vi "Register for Sequence Complete Event.vi"(8 "error in (no error)":errorcluster, 10 "Sequence Names":string[](array[string]), 11 "Session Ref in":T2) -> (0 "error out":errorcluster, 1 "Event Registration Refnum":refnum<event-registration>, 2 "Sequence Names out":string[](array[string]), 3 "Session Ref out":T2, 5 "Sequence Complete Event Ref":T1)   [LabVIEW 2020, in "NI_VS Sequence Execution Interface.lvlib"]
doc: "Registers for a sequence complete event for the set of sequences you specify. A sequence complete event is triggered when a sequence completes execution. This VI returns a registered user event reference and information about the event."
uses:
  <vilib>/NI VeriStand/Execution/SequenceExecutionInterface/NI_VS Sequence Execution Interface.lvlib
  <vilib>/NI VeriStand/Execution/SequenceExecutionInterface/Stimulus Profile Session Ref.ctl
  NationalInstruments.VeriStand.ClientAPI
  <vilib>/NI VeriStand/Execution/SequenceExecutionInterface/Sequence Complete Event Ref.ctl
  <vilib>/NI VeriStand/Execution/SequenceExecutionInterface/Sequence Complete Event Data.ctl
  <vilib>/NI VeriStand/Execution/SequenceExecutionInterface/Data Value Ref.ctl
  NationalInstruments.VeriStand.DataTypes
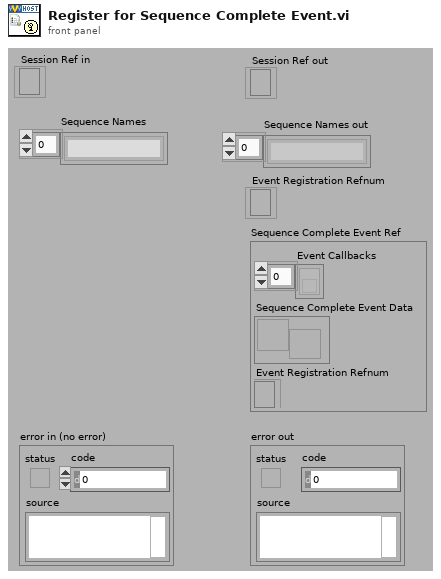
[diagram p1: front panel]
types:
  T1 = typedef "NI_VS Sequence Execution Interface.lvlib/Sequence Complete Event Ref.ctl" = cluster{"Event Callbacks":refnum<k27>[], "Sequence Complete Event Data":refnum<user-event>, "Event Registration Refnum":refnum<event-registration>}
  T2 = typedef "NI_VS Sequence Execution Interface.lvlib/Stimulus Profile Session Ref.ctl" = refnum<k24>
  T3 = typedef "NI_VS Sequence Execution Interface.lvlib/Sequence Complete Event Data.ctl" = cluster{"Sequence Name":string, "Return Value":T4, "Aborted":bool, "Error":errorcluster}
  T4 = typedef "NI_VS Sequence Execution Interface.lvlib/Data Value Ref.ctl" = refnum<k24>
  T5 = cluster{refnum<k27>[], "Sequence Complete Event Data":refnum<user-event>, "Event Registration Refnum":refnum<event-registration>}
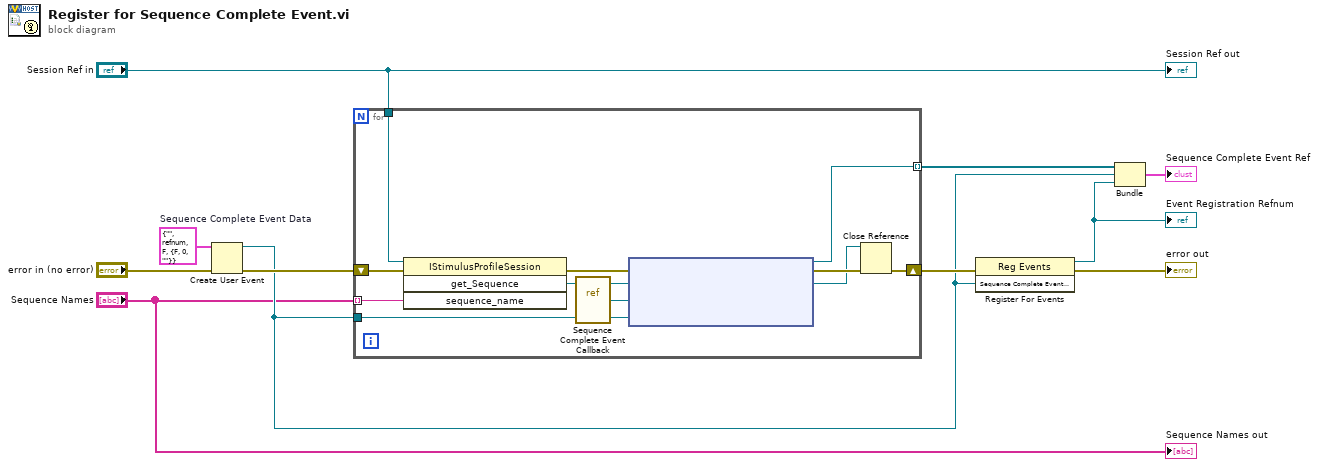
[diagram p0: block diagram]
diagram:
  w4 = T3 {"Sequence Name"="", "Return Value"=refnum, "Aborted"=FALSE, "Error"={"status"=FALSE, "code"=0, "source"=""}}  # Sequence Complete Event Data
  n1 = Create User Event(user event datatype=w4, error in="error in (no error)") -> (user event=w7:refnum<user-event>, error out=w11:errorcluster)
  n2 = for {
    tunnel: [w19] -> w9 mode=indexing
    tunnel: w7 -> [w18]
    tunnel: "Session Ref in" -> [w17]
    tunnel: "Sequence Names" -> [w14] mode=indexing
    shift-right: [w20] -> w10
    shift-left: w11 -> [w21]
    n3 = invoke class="IStimulusProfileSession" method="get_Sequence"(reference=w17, error in=w21, "sequence_name"=w14) -> (error out=w12:errorcluster, "get_Sequence"=w15:refnum<k24>)  [unwired: 1 in, 2 out]
    n4 = vi-ref <vilib>:"Sequence Complete Event Callback.vi"() -> ("vi reference"=w13:refnum<vi>)
    n5 = node(w12, w15, w13, w18) -> (w19:refnum<k27>, w16:errorcluster)  [unwired: 1 in]
    n6 = Close Reference(reference=w15, error in (no error)=w16) -> (error out=w20:errorcluster)
  }
  n7 = register-events(error in=w10, w7) -> (reference out=w1:refnum<event-registration>, error out=→"error out":errorcluster)  [unwired: 1 in]
  "Event Registration Refnum" <- w1
  n8 = Bundle(w9, "Sequence Complete Event Data"=w7, "Event Registration Refnum"=w1) -> (→"Sequence Complete Event Ref":T5)  [unwired: 1 in]
  "Session Ref out" <- "Session Ref in"
  "Sequence Names out" <- "Sequence Names"
